vi "TCP Multiple Connections - Server.vi"() -> ()   [LabVIEW 2015]
doc: "This is the TCP server VI that supports multiple connections from client VIs."
uses:
  controls/TCP Multiple Connections State.ctl
  controls/TCP Multiple Connections Data.ctl
panel:
  in  "Stop":bool
  out "Current Data":dbl
  out "# of Connections":i32
  # "Overview: Demonstrates the use of the TCP functions to initialize a TCP server that can send data to multiple client VIs.\nInstructions:\n1. Run the VI.\n2. Open TCP Multiple Connections - Client 1.vi and follow the instructions on its front panel.\n3. Open TCP Multiple Connections - Client 2.vi and follow the instructions on its front panel.\n4. Click Stop to stop the VI."
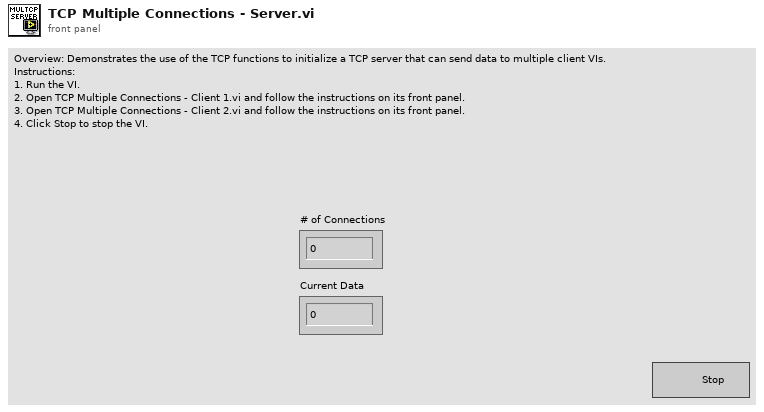
[diagram p1: front panel]
types:
  T1 = typedef "TCP Multiple Connections Data.ctl" = cluster{"Clients":refnum<k5>[], "Listener":refnum<k5>}
  T2 = typedef "TCP Multiple Connections State.ctl" = enum16{"Initialize", "Status Check", "Send Data", "Stop"}
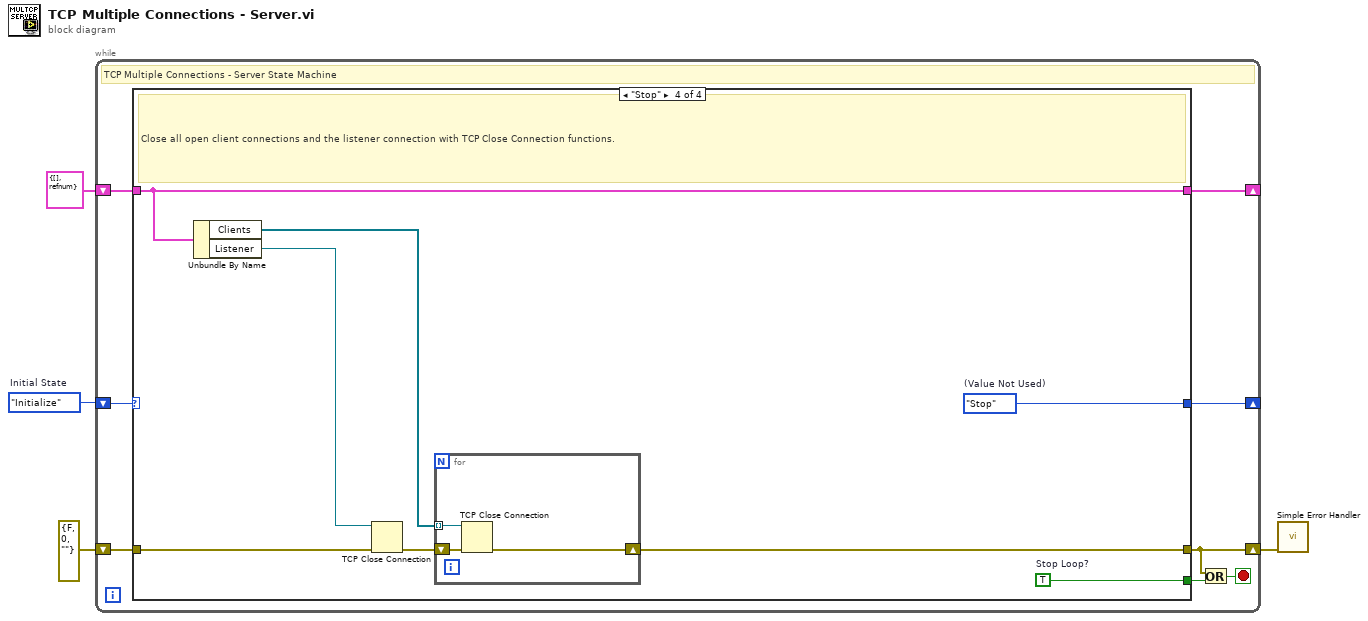
[diagram p0: block diagram]
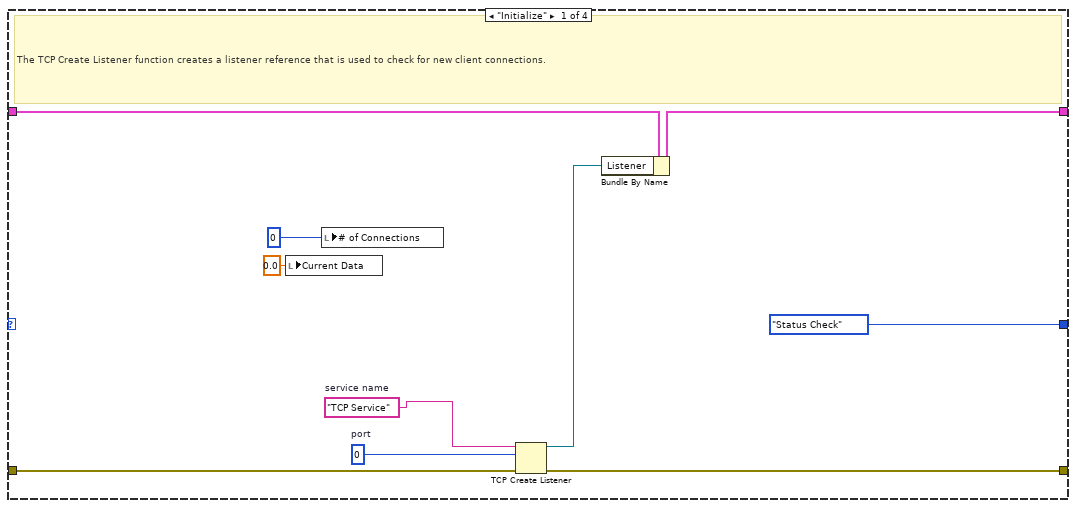
[diagram p2: hidden frame]
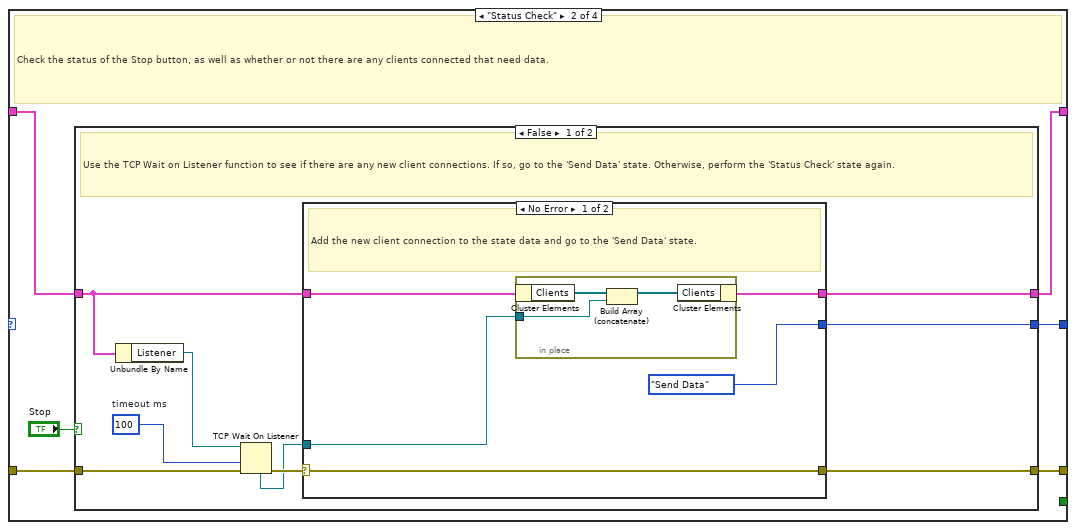
[diagram p3: hidden frame]
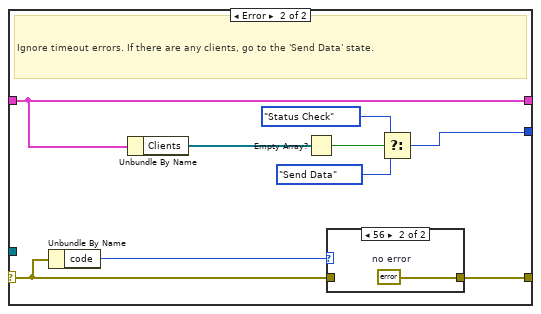
[diagram p4: hidden frame]
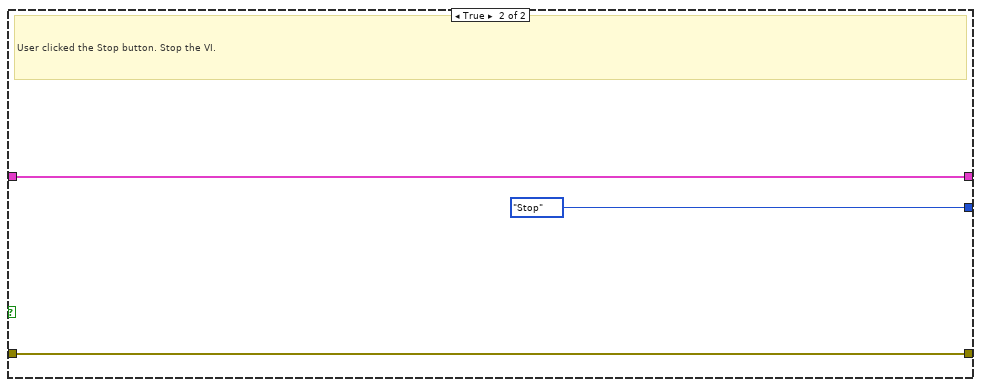
[diagram p6: hidden frame]
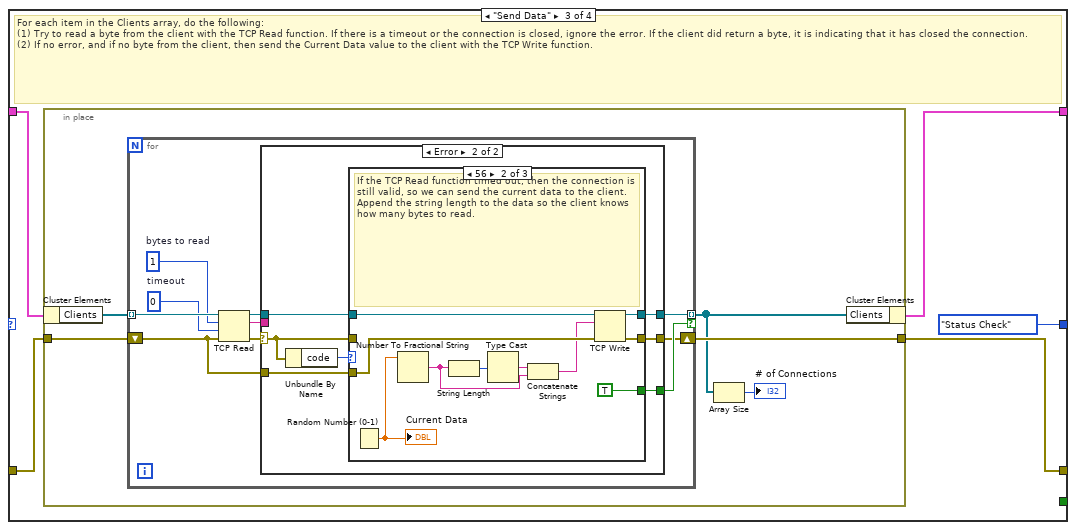
[diagram p7: hidden frame]
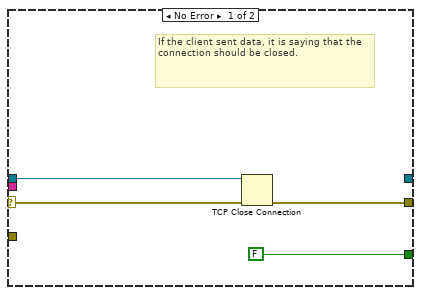
[diagram p8: hidden frame]
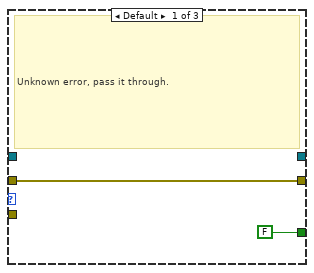
[diagram p9: hidden frame]
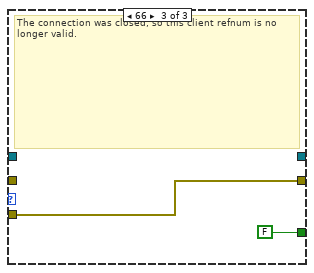
[diagram p10: hidden frame]
diagram:
  w4 = TCP_Multiple_Connections_State."Initialize"  # Initial State
  n1 = while {
    shift-right: [w11] -> _
    shift-left: w4 -> [w12]
    shift-right: [w9] -> _
    shift-left: T1 {"Clients"=[], "Listener"=refnum} ("Data") -> [w10]
    shift-right: [w5] -> w1
    shift-left: errorcluster {"status"=FALSE, "code"=0, "source"=""} ("error constant") -> [w8]
    stop <- w6 stop-if-true
    # "TCP Multiple Connections - Server State Machine"
    n2 = case shown="\"Stop\"" w12 {
      tunnel: [TCP_Multiple_Connections_State."Status Check" ("States") w28 TCP_Multiple_Connections_State."Status Check" ("States") w105] -> w11
      tunnel: [_ _ _ w112] -> w7
      tunnel: w10 -> [w20 w24 w62 w111]
      tunnel: [w13 w23 w61 w111] -> w9
      tunnel: w8 -> [w22 w27 w64 w110]
      tunnel: [w21 w26 w63 w108] -> w5
      frame "Initialize" {
        w15 = "TCP Service"  # service name
        w14 = u16 0  # port
        # "The TCP Create Listener function creates a listener reference that is used to check for new client connections."
        n3 = local write "Current Data"(0.0 ("Current Data")) -> ()
        n4 = local write "# of Connections"(0 ("Number of Client Connections")) -> ()
        n5 = TCP Create Listener(8:w22, 10:w14, 11:w15) -> (0:w21:errorcluster, 3:w19:refnum<k5>)  [unwired: 3 out]
        n6 = Bundle By Name(cluster=w20, "Listener"=w19) -> (w13:T1)
      }
      frame "Status Check" {
        # "Check the status of the Stop button, as well as whether or not there are any clients connected that need data."
        n7 = case shown="False" "Stop" {
          tunnel: [w37 TCP_Multiple_Connections_State."Stop" ("States")] -> w28
          tunnel: w27 -> [w36 w59]
          tunnel: [w29 w59] -> w26
          tunnel: w24 -> [w32 w58]
          tunnel: [w31 w58] -> w23
          frame False {
            w35 = 100  # timeout ms
            # "Use the TCP Wait on Listener function to see if there are any new client connections. If so, go to the 'Send Data' state. Otherwise, perform the 'Status Check' state again."
            n8 = Unbundle By Name(w32) -> ("Listener"=w30:refnum<k5>)
            n9 = TCP Wait On Listener(8:w36, 9:w35, 11:w30) -> (0:w34:errorcluster, 4:w33:refnum<k5>)  [unwired: 4 out]
            n10 = case shown="No Error" w34 {
              selector: w34 -> [w40 w54]
              tunnel: [TCP_Multiple_Connections_State."Send Data" ("States") w48] -> w37
              tunnel: w33 -> [w41 _]
              tunnel: w32 -> [w42 w51]
              tunnel: [w39 w51] -> w31
              tunnel: [w40 w52] -> w29
              frame No Error {
                # "Add the new client connection to the state data and go to the 'Send Data' state."
                n11 = in-place {
                  in-place-border: w41 -> [w43]
                  n12 = in-place-cluster #1(w42) -> ("Clients"=w45:refnum<k5>[])
                  n13 = Build Array (concatenate)(w45, w43) -> (w44:refnum<k5>[])
                  n14 = in-place-cluster #1("Clients"=w44) -> (w39:T1)
                }
              }
              frame Error {
                # "Ignore timeout errors. If there are any clients, go to the 'Send Data' state."
                n15 = Unbundle By Name(w54) -> ("code"=w53:i32)
                n16 = Unbundle By Name(w51) -> ("Clients"=w50:refnum<k5>[])
                n17 = Empty Array?(array=w50) -> (empty?=w49:bool)
                n18 = case shown="56" w53 {
                  tunnel: w54 -> [w55 _]
                  tunnel: [w55 w56] -> w52
                  frame Default {
                  }
                  frame 56 {
                    w56 = errorcluster {"status"=FALSE, "code"=0, "source"=""}  # no error
                  }
                }
                n19 = Select(t=TCP_Multiple_Connections_State."Status Check" ("States"), s=w49, f=TCP_Multiple_Connections_State."Send Data" ("States")) -> (s? t:f=w48:T2)
              }
            }
          }
          frame True {
            # "User clicked the Stop button. Stop the VI."
          }
        }
      }
      frame "Send Data" {
        # "For each item in the Clients array, do the following:\n(1) Try to read a byte from the client with the TCP Read function. If there is a timeout or the connection is closed, ignore the error. If the client did return a byte, it is indicating that it has closed the connection.\n(2) If no error, and if no byte from the client, then send the Current Data value to the client with the TCP Write function."
        n20 = in-place {
          in-place-border: w64 -> [w69]
          in-place-border: [w68] -> w63
          n21 = in-place-cluster #2(w62) -> ("Clients"=w66:refnum<k5>[])
          n22 = for {
            tunnel: w66 -> [w79] mode=indexing
            shift-right: [w71] -> w68
            shift-left: w69 -> [w70]
            tunnel: [w73] -> w65 mode=indexing if=w72
            w76 = 0  # timeout
            w77 = 1  # bytes to read
            n23 = TCP Read(connection ID=w79, bytes to read=w77, error in (no error)=w70, 9:w76) -> (connection ID out=w78:refnum<k5>, data out=w74:string, error out=w75:errorcluster)  [unwired: 1 out]
            n24 = case shown="Error" w75 {
              selector: w75 -> [w82 w89]
              tunnel: w78 -> [w83 w86]
              tunnel: w74 -> [_ _]
              tunnel: [_ w84] -> w73
              tunnel: [FALSE w85] -> w72
              tunnel: [w80 w88] -> w71
              tunnel: w70 -> [_ w87]
              frame No Error {
                # "If the client sent data, it is saying that the connection should be closed."
                # "If the client sent data, it is saying that the connection should be closed."
                n25 = TCP Close Connection(connection ID=w83, error in (no error)=w82) -> (error out=w80:errorcluster)  [unwired: 2 out]
              }
              frame Error {
                # "Ignore connection closed and timeout errors"
                n26 = Unbundle By Name(w89) -> ("code"=w90:i32)
                n27 = case shown="56" w90 {
                  tunnel: w89 -> [w92 _ _]
                  tunnel: [w92 w102 w104] -> w88
                  tunnel: w87 -> [_ w98 w104]
                  tunnel: w86 -> [_ w101 _]
                  tunnel: [FALSE TRUE FALSE] -> w85
                  tunnel: [_ w100 _] -> w84
                  frame Default {
                    # "Unknown error, pass it through."
                  }
                  frame 56 {
                    # "If the TCP Read function timed out, then the connection is still valid, so we can send the current data to the client. Append the string length to the data so the client knows how many bytes to read."
                    n28 = Random Number (0-1)() -> (number: 0 to 1=w97:dbl)
                    "Current Data" <- w97
                    n29 = Number To Fractional String(number=w97) -> (F-format string=w94:string)  [unwired: 3 in]
                    n30 = String Length(string=w94) -> (length=w95:i32)
                    n31 = Type Cast(x=w95) -> (*(type *) &x=w96:string)  [unwired: 1 in]
                    n32 = Concatenate Strings(w96, w94) -> (w93:string)
                    n33 = TCP Write(connection ID=w101, data in=w93, error in (no error)=w98) -> (connection ID out=w100:refnum<k5>, error out=w102:errorcluster)  [unwired: 2 out]
                  }
                  frame 66 {
                    # "The connection was closed, so this client refnum is no longer valid."
                  }
                }
              }
            }
          }
          n34 = Array Size(array=w65) -> (size(s)=→"# of Connections":i32)
          n35 = in-place-cluster #2("Clients"=w65) -> (w61:T1)
        }
      }
      frame "Stop" {
        w105 = TCP_Multiple_Connections_State."Stop"  # (Value Not Used)
        w112 = TRUE  # Stop Loop?
        # "Close all open client connections and the listener connection with TCP Close Connection functions."
        n36 = Unbundle By Name(w111) -> ("Clients"=w109:refnum<k5>[], "Listener"=w106:refnum<k5>)
        n37 = TCP Close Connection(connection ID=w106, error in (no error)=w110) -> (error out=w107:errorcluster)  [unwired: 1 in, 1 out]
        n38 = for {
          shift-right: [w114] -> w108
          shift-left: w107 -> [w115]
          tunnel: w109 -> [w113] mode=indexing
          n39 = TCP Close Connection(connection ID=w113, error in (no error)=w115) -> (error out=w114:errorcluster)  [unwired: 1 in, 1 out]
        }
      }
    }
    n40 = Or(x=w5, y=w7) -> (x .or. y?=w6:bool)
  }
  n41 = call <vilib>:"Simple Error Handler.vi"("error in (no error)"=w1) -> ()  [unwired: 4 in, 5 out]
